vi "Display.vi"(8 "error in":errorcluster, 11 "Input (I32) in":refnum<class "SVG - Input (I32).lvclass">) -> (0 "error out":errorcluster, 3 "Input (I32) out":refnum<class "SVG - Input (I32).lvclass">)   [LabVIEW 2021, in "SVG - Input (I32).lvclass"]
doc: "This vi will display the input pop up waiting for a type I32 input from the user and will show a customized image.\n\n<b>Code Developed By:</b>\nDaniel Coons\nTechnology Service Corporation\n1983 S Liberty Drive\nBloomington, IN 47403\nPhone: 812 558-7100\ndaniel.coons@tsc.com\nwww.tsc.com/atcs"
uses:
  SVG - Input (I32).lvclass
  C:/Program Files (x86)/National Instruments/LabVIEW 2021/vi.lib/addons/_TSC/TSC Pop-Up/Popup/Popup.lvclass
  SVG - Input (I32).lvclass/SVG - Input (I32).ctl
  <vilib>/addons/_TSC/TSC Pop-Up/Popup/Popup.lvclass/Popup.ctl
  <vilib>/addons/_TSC/TSC Pop-Up/Popup/Data Member Access/Read Theme.vi
  <vilib>/addons/_TSC/TSC Pop-Up/Theme/Theme.lvclass
  <vilib>/addons/_TSC/TSC Pop-Up/Popup/Popup.lvclass
  user32.dll
panel:
  out "header":bool
  in  "OK":bool
  in  "Input":i32
  out "Input value out":i32=1 min=1
  out "2D Picture":picture
  out "Message":string
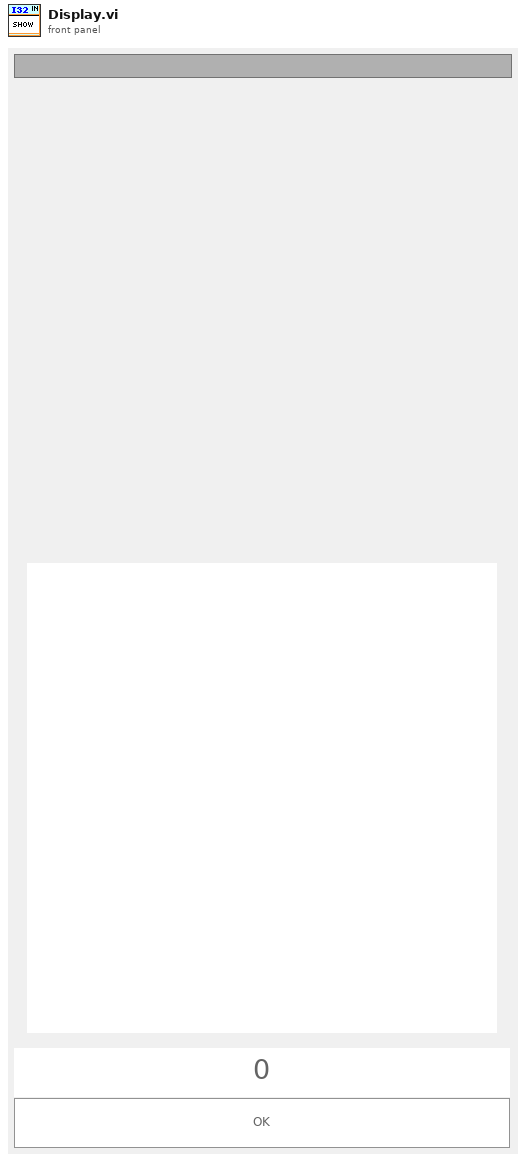
[diagram p1: front panel]
types:
  T1 = typedef "LVPoint32TypeDef.ctl" = cluster{"Horizontal":i32, "Vertical":i32}
  T2 = typedef "LVPositionTypeDef.ctl" = cluster{"Left":i32, "Top":i32}
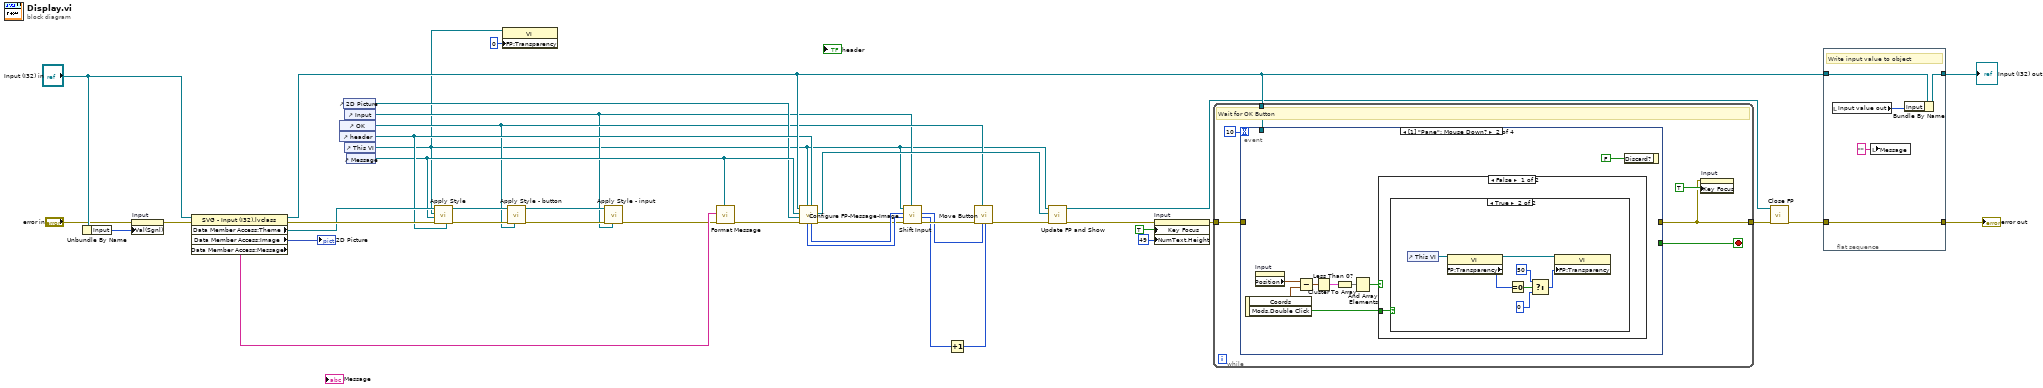
[diagram p0: block diagram]
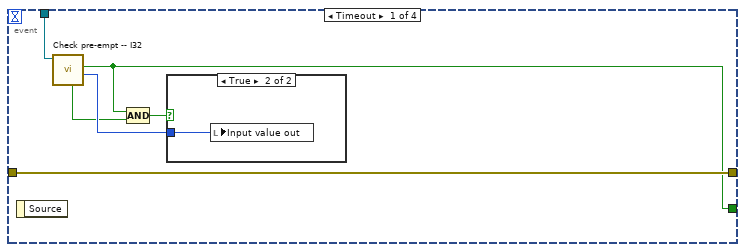
[diagram p2: hidden frame]
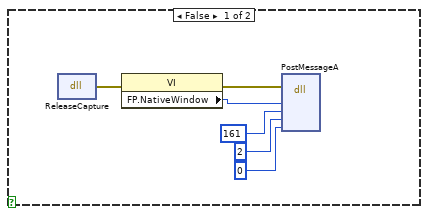
[diagram p4: hidden frame]
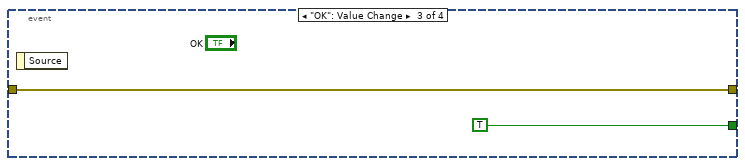
[diagram p6: hidden frame]
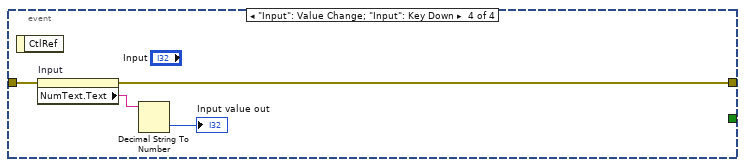
[diagram p7: hidden frame]
diagram:
  n1 = Unbundle By Name("Input (I32) in") -> ("Input"=w35:i32)
  n2 = property on="Input" class="DigNum (strict)"(error in="error in", "Val(Sgnl)"=w35) -> (error out=w36:errorcluster)  [unwired: 1 in, 1 out]
  n3 = property class="SVG - Input (I32).lvclass"(reference="Input (I32) in", error in=w36) -> (reference out=w19:refnum<class "SVG - Input (I32).lvclass">, error out=w34:errorcluster, "Data Member Access:Theme"=w24:refnum<class "Theme.lvclass">, "Data Member Access:Image"=→"2D Picture":picture, "Data Member Access:Message"=w26:string)
  n4 = control-ref of="OK"() -> (w6:refnum<vi>)
  n5 = control-ref of="header"() -> (w18:refnum<vi>)
  n6 = control-ref of="2D Picture"() -> (w16:refnum<vi>)
  n7 = control-ref of="Input"() -> (w5:refnum<vi>)
  n8 = control-ref of="This VI"() -> (w1:refnum<vi>)
  n9 = control-ref of="Message"() -> (w17:refnum<vi>)
  n10 = call <vilib>:"Apply Style.vi"("header ref"=w18, "error in (no error)"=w34, "message ref"=w17, "pop up ref"=w1, "Theme in"=w24) -> ("error out"=w25:errorcluster, "Theme out"=w21:refnum<class "Theme.lvclass">)  [unwired: 5 in]
  n11 = property on="Property Node" class="VI"(reference=w1, "FP:Transparency"=u8 0 ("Front Panel Window:Transparency")) -> ()  [unwired: 1 in, 2 out]
  n12 = call <vilib>:"Apply Style - button.vi"("button ref"=w6, "error in (no error)"=w25, "Theme in"=w21) -> ("error out"=w23:errorcluster, "Theme out"=w20:refnum<class "Theme.lvclass">)  [unwired: 7 in]
  n13 = call <vilib>:"Apply Style - input.vi"("input ref"=w5, "error in (no error)"=w23, "Theme in"=w20) -> ("error out"=w22:errorcluster)  [unwired: 7 in, 1 out]
  n14 = call <vilib>:"Format Message.vi"("formatted string"=w17, "error in"=w22, "String Input"=w26) -> ("error out"=w27:errorcluster)  [unwired: 7 in, 1 out]
  n15 = call <vilib>:"Configure FP-Message-Image.vi"("header ref"=w18, "Pop Up ref"=w1, "error in (no error)"=w27, "Image ref"=w16, "Message ref"=w17, "Popup in"=w19) -> ("error out"=w8:errorcluster, "Panel Ref"=w7:refnum<vi>, "Panel Width"=w10:i32, "Panel Height"=w9:i32)  [unwired: 1 in, 1 out]
  n16 = call <vilib>:"Shift Input.vi"("Control"=w5, "Error In"=w8, "Panel Height"=w9, "Panel Width"=w10, "Pop Up ref"=w1) -> ("Error Out"=w15:errorcluster, "Panel Height out"=w13:i32, "Panel Width out"=w14:i32)  [unwired: 4 in]
  n17 = Increment(x=w13) -> (x+1=w12:i32)
  n18 = call <vilib>:"Move Button.vi"("Panel Height"=w12, "Panel Width"=w14, "Button"=w6, "Error In"=w15) -> ("Error Out"=w11:errorcluster)  [unwired: 6 in, 1 out]
  n19 = call <vilib>:"Update FP and Show.vi"("error in (no error)"=w11, "Panel Ref"=w7, "VI in"=w1) -> ("error out"=w31:errorcluster, "VI out"=w4:refnum<vi>)  [unwired: 7 in]
  n20 = property on="Input" class="DigNum (strict)"(error in=w31, "Key Focus"=TRUE, "NumText.Height"=u32 49 ("Numeric Text.Size:Height")) -> (error out=w30:errorcluster)  [unwired: 1 in, 1 out]
  n21 = while {
    tunnel: w30 -> [w46]
    tunnel: [w41] -> w33
    tunnel: w19 -> [w43]
    stop <- w45 stop-if-true
    # "Wait for OK Button"
    n22 = event shown="[1] \"Pane\": Mouse Down?" {
      selector: _ -> [_ _ _ _]
      dyn-events: _ -> [_ _ _ _]
      timeout: 10 -> [_ _ _ _]
      tunnel: w46 -> [w49 _ w77 w81]
      tunnel: [w49 _ w77 w79] -> w41
      tunnel: [w48 _ TRUE _] -> w45
      tunnel: w43 -> [w47 _ _ _]
      event Timeout {
        n23 = event-data() -> ()  [unwired: 1 in, 1 out]
        n24 = call <vilib>:"Check pre-empt -- I32.vi"("_Popup in"=w47) -> ("Value?"=w52:i32, "Pre-empted?"=w48:bool, "Type Match?"=w50:bool)  [unwired: 7 in, 1 out]
        n25 = Compound Arithmetic op=AND(w48, w50) -> (w51:bool)
        n26 = case shown="True" w51 {
          tunnel: w52 -> [_ w53]
          frame False {
          }
          frame True {
            n27 = local write "Input value out"(w53) -> ()
          }
        }
      }
      event Mouse Down? {
        n28 = event-data() -> ("Coords"=w55:T1, "Mods.Double Click"=w54:bool)  [unwired: 1 in]
        n29 = property on="Input" class="DigNum (strict)"() -> ("Position"=w56:T2)  [unwired: 2 in, 2 out]
        n30 = Subtract(x=w56, y=w55) -> (x-y=w57:T2)
        n31 = Less Than 0?(x=w57) -> (x < 0?=w58:cluster{"Left":bool, "Top":bool})
        n32 = Cluster To Array(cluster=w58) -> (array=w59:bool[])
        n33 = And Array Elements(Boolean array=w59) -> (logical AND=w60:bool)
        n34 = case shown="False" w60 {
          tunnel: w54 -> [w62 _]
          frame False {
            n35 = case shown="True" w62 {
              frame False {
                n36 = dll-call lib="user32.dll" fn="ReleaseCapture"() -> (error out=w66:errorcluster)  [unwired: 4 in, 1 out]
                n37 = property class="VI"(error in=w66) -> (error out=w67:errorcluster, "FP.NativeWindow"=w68:u64)  [unwired: 1 in, 1 out]
                n38 = dll-call lib="user32.dll" fn="PostMessageA"(error in=w67, "hWnd"=w68, "Msg"=161, "wParam"=2, "lParam"=0) -> ()  [unwired: 7 in, 2 out]
              }
              frame True {
                n39 = control-ref of="This VI"() -> (w75:refnum<vi>)
                n40 = property class="VI"(reference=w75) -> (reference out=w73:refnum<vi>, "FP:Transparency"=w74:u8)  [unwired: 1 in, 1 out]
                n41 = Equal To 0?(x=w74) -> (x = 0?=w72:bool)
                n42 = Select(t=u8 50, s=w72, f=u8 0) -> (s? t:f=w71:u8)
                n43 = property class="VI"(reference=w73, "FP:Transparency"=w71) -> ()  [unwired: 1 in, 2 out]
              }
            }
          }
          frame True {
          }
        }
        n44 = event-data("Discard?"=FALSE) -> ()  [unwired: 1 in, 1 out]
      }
      event "OK": Value Change {
        n45 = event-data() -> ()  [unwired: 1 in, 1 out]
      }
      event "Input": Value Change; "Input": Key Down {
        n46 = event-data() -> ()  [unwired: 1 in, 1 out]
        n47 = property on="Input" class="DigNum (strict)"(error in=w81) -> (error out=w79:errorcluster, "NumText.Text"=w80:string)  [unwired: 1 in, 1 out]
        n48 = Decimal String To Number(string=w80) -> (number=→"Input value out":i32)  [unwired: 2 in, 1 out]
      }
    }
    n49 = property on="Input" class="DigNum (strict)"(error in=w41, "Key Focus"=TRUE) -> ()  [unwired: 1 in, 2 out]
  }
  n50 = call <vilib>:"Close FP.vi"("error in (no error)"=w33, "VI in"=w4) -> ("error out"=w32:errorcluster)  [unwired: 9 in]
  n51 = flat-sequence {
    tunnel: w32 -> [w86]
    tunnel: [w86] -> w37
    tunnel: w19 -> [w85]
    tunnel: [w84] -> w38
    frame #0 {
      # "Write input value to object"
      n52 = local read "Input value out"() -> (w83:i32)
      n53 = local write "Message"("" ("Message")) -> ()
      n54 = Bundle By Name(cluster=w85, "Input"=w83) -> (w84:refnum<class "SVG - Input (I32).lvclass">)
    }
  }
  "error out" <- w37
  "Input (I32) out" <- w38
